vi "Apply DSF Configuration to Node.vi"(8 "error in (no error)":errorcluster, 10 "configuration path":path, 11 "Item Ref in":T1 format="%.0x") -> (0 "error out":errorcluster)   [LabVIEW 2020, in "DSF System Explorer.lvlib"]
uses:
  DSF System Explorer.lvlib
  <vilib>/NI VeriStand/Custom Device API/Custom Device Item Ref.ctl
  Includes/DSF Core.lvlibp/Classes/Configuration Session/Configuration Session.lvclass
  <vilib>/NI VeriStand/Custom Device API/Custom Device API.lvlib
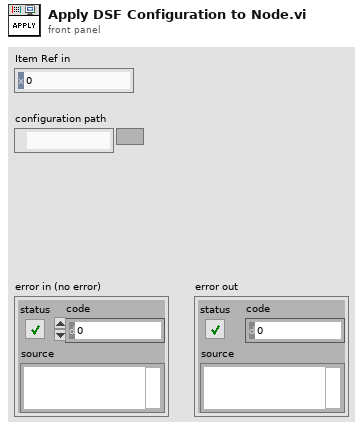
[diagram p1: front panel]
types:
  T1 = typedef "Custom Device API.lvlib/Custom Device Item Ref.ctl" = u64
  T2 = typedef "DSF Core.lvlibp/DSF Version Info.ctl" = cluster{"major":u32, "minor":u32, "fix":u32, "build":string}
  T3 = typedef "DSF Core.lvlibp/DSF Engine Framework Configuration.ctl" = cluster{"plugins":T4[]}
  T4 = typedef "DSF Core.lvlibp/DSF Engine Plugin Configuration.ctl" = cluster{"core":T5, "component settings":T7[], "threads":T8[]}
  T5 = typedef "DSF Core.lvlibp/Plugin Configuration.lvclass/Core Plugin Configuration.ctl" = cluster{"name":string, "components":string[], "cycle timing":T6}
  T6 = typedef "DSF Core.lvlibp/DSF Timing Info.ctl" = cluster{"priority":u64, "decimation":u64, "offset":u64}
  T7 = typedef "DSF Core.lvlibp/DSF Settings Info.ctl" = cluster{"component":string, "values":cluster{"key":string, "value":string}[]}
  T8 = typedef "DSF Core.lvlibp/DSF Engine Plugin Thread Configuration.ctl" = cluster{"core":T9, "component settings":T7[], "transfer groups":T10[]}
  T9 = typedef "DSF Core.lvlibp/Thread Configuration.lvclass/Core Thread Configuration.ctl" = cluster{"processor":i32, "priority offset":i16}
  T10 = typedef "DSF Core.lvlibp/DSF Engine Transfer Group Configuration.ctl" = cluster{"core":T11, "component settings":T7[], "transfers":T14[]}
  T11 = typedef "DSF Core.lvlibp/Group Configuration.lvclass/Core Group Configuration.ctl" = cluster{"name":string, "direction":T12, "cycle timing":T6, "timeout behavior":T13, "enable conversion":bool}
  T12 = typedef "DSF Core.lvlibp/DSF Direction.ctl" = enum8{"Tx", "Rx"}
  T13 = typedef "DSF Core.lvlibp/DSF Timeout Behavior.ctl" = enum8{"Increment Late Count", "Throw Error"}
  T14 = typedef "DSF Core.lvlibp/DSF Engine Transfer Configuration.ctl" = cluster{"core":T15, "component settings":T7[], "channels":T16[]}
  T15 = typedef "DSF Core.lvlibp/Transfer Configuration.lvclass/Core Transfer Configuration.ctl" = cluster{"name":string}
  T16 = typedef "DSF Core.lvlibp/DSF Engine Channel Configuration.ctl" = cluster{"core":T17, "component settings":T7[]}
  T17 = typedef "DSF Core.lvlibp/Channel Configuration.lvclass/Core Channel Configuration.ctl" = cluster{"name":string, "units":string, "engine data type":T18, "string data type":T18, "string offset":u64}
  T18 = typedef "DSF Core.lvlibp/DSF Data Type.ctl" = enum8{"Bool", "SGL", "DBL", "I8", "I16", "I32", "I64", "U8", "U16", "U32", "U64"}
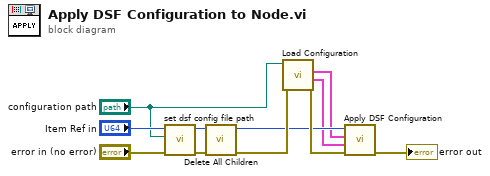
[diagram p0: block diagram]
diagram:
  n1 = call "set dsf config file path.vi"("error in (no error)"="error in (no error)", "Path"="configuration path", "Item Ref in"="Item Ref in") -> ("error out"=w9:errorcluster, "Item Ref out"=w10:T1)  [unwired: 7 in]
  n2 = call "Delete All Children.vi"("error in (no error)"=w9, "Item Ref in"=w10) -> ("error out"=w6:errorcluster, "Item Ref out"=w5:T1)  [unwired: 8 in]
  n3 = call "Load Configuration.vi"("error in (no error)"=w6, "configuration file path"="configuration path") -> ("error out"=w7:errorcluster, "version"=w2:T2, "framework configuration"=w3:T3)  [unwired: 6 in, 1 out]
  n4 = call "Apply DSF Configuration.vi"("error in (no error)"=w7, "version"=w2, "framework configuration"=w3, "Item Ref in"=w5) -> ("error out"=→"error out":errorcluster)  [unwired: 7 in]
